vi "sweep_finished.vi"(8 "error in (no error)":errorcluster, 11 "DataCollectionMG091001IntrinsicImaging in":refnum<class "DataCollectionMG091001IntrinsicImaging.lvclass">) -> (0 "error out":errorcluster, 3 "DataCollectionMG091001IntrinsicImaging out":refnum<class "DataCollectionMG091001IntrinsicImaging.lvclass">)   [LabVIEW 2010, in "DataCollectionMG091001IntrinsicImaging.lvclass"]
uses:
  DataCollectionMG091001IntrinsicImaging.lvclass
  DataCollectionMG091001IntrinsicImaging.lvclass/DataCollectionMG091001IntrinsicImaging.ctl
  ExperimentController/GenericExperimentController/GenericExperimentController/trigger_enum.ctl
  ExperimentController/GenericExperimentController/GenericExperimentController/GenericExperimentController.lvclass
  common/classes/GenericComponent/GenericComponent/class_data.vi
  common/classes/GenericComponent/GenericComponent/GenericComponent.lvclass
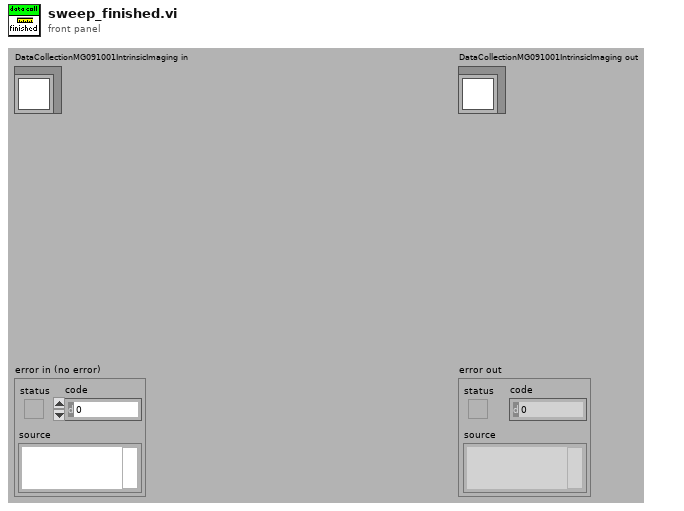
[diagram p1: front panel]
types:
  T1 = typedef "GenericExperimentController.lvclass/trigger_enum.ctl" = enum16{"NULL", "proceed", "prepare"}
  T2 = typedef "DataCollectionMG091001IntrinsicImaging.lvclass/individual_sweeps_saving_enum.ctl" = enum32{"autosave sweeps on the fly", "save individual sweeps", "don't save individual sweeps"}
  T3 = typedef "run_mode_enum.ctl" = enum16{"focus mode", "single sweep mode", "experiment mode"}
  T4 = typedef "main_trigger_enum.ctl" = enum16{"NULL", "initialise", "terminate", "start", "stop", "change objective", "change experimentController", "change imagingMode", "save notebook", "started saving", "finished saving", "expCtr ready", "expCtr missing", "imgMd ready", "imgMd missing", "scanHd ready", "scanHd missing", "DAQ ready", "DAQ missing", "imgAsm ready", "imgAsm missing", "dataColl ready", "dataColl missing", "display ready", "display missing", "analysr ready", "analysr missing", "instrmnt ready", "instrmnt missing", "stimltr ready", "stimltr missing", "stage ready", "stage missing"}
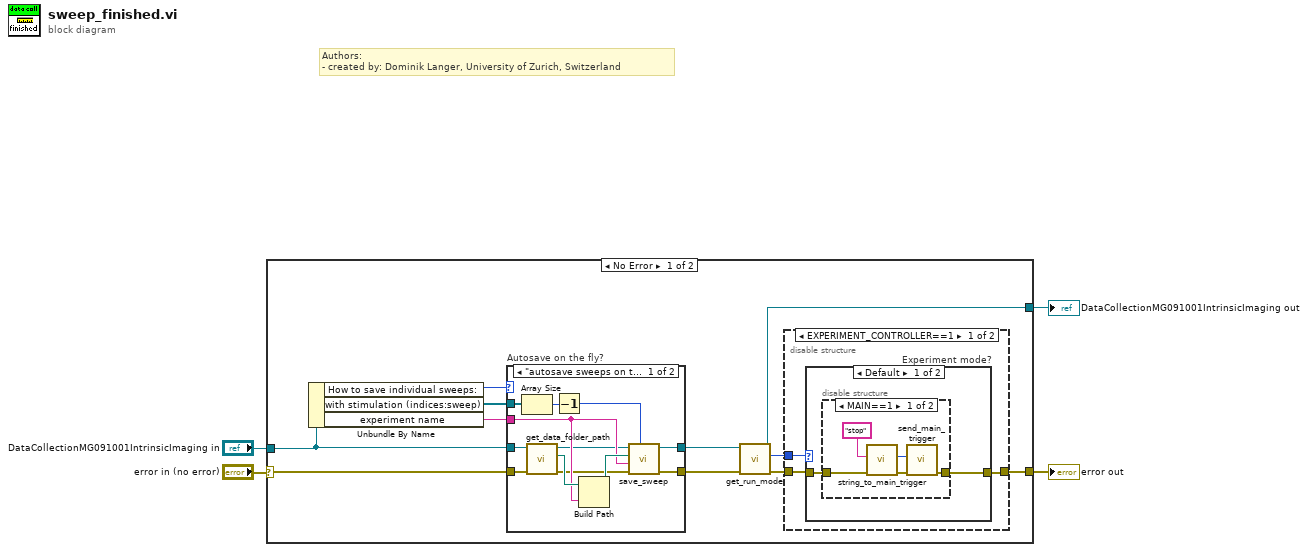
[diagram p0: block diagram]
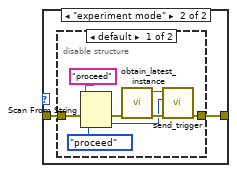
[diagram p3: hidden frame]
diagram:
  # "Authors: \n- created by: Dominik Langer, University of Zurich, Switzerland"
  n1 = case shown="No Error" "error in (no error)" {
    selector: "error in (no error)" -> [w11 w53]
    tunnel: "DataCollectionMG091001IntrinsicImaging in" -> [w12 w54]
    tunnel: [w8 w53] -> w2
    tunnel: [w5 w54] -> w1
    frame No Error {
      n2 = Unbundle By Name(w12) -> ("How to save individual sweeps:"=w13:T2, "with stimulation (indices:sweep)"=w14:refnum<class "ImageCollection.lvclass">[], "experiment name"=w15:string)
      n3 = case "Autosave on the fly?" shown="\"autosave sweeps on the fly\"" w13 {
        tunnel: [w50 w52] -> w6
        tunnel: [w49 w51] -> w7
        tunnel: w12 -> [w48 w52]
        tunnel: w11 -> [w47 w51]
        tunnel: w15 -> [w44 _]
        tunnel: w14 -> [w41 _]
        frame "autosave sweeps on the fly" {
          n4 = Array Size(array=w41) -> (size(s)=w40:i32)
          n5 = call-dynamic "get_data_folder_path.vi"("error in (no error)"=w47, "GenericComponent in"=w48) -> ("error out"=w43:errorcluster, "data folder path"=w46:path, "GenericComponent out"=w42:refnum<class "DataCollectionMG091001IntrinsicImaging.lvclass">)  [unwired: 7 in]
          n6 = Decrement(x=w40) -> (x-1=w39:i32)
          n7 = Build Path(base path=w46, name or relative path=w44) -> (appended path=w45:path)
          n8 = call-dynamic "save_sweep.vi"("sweep index"=w39, "error in (no error)"=w43, "base name"=w44, "folder path"=w45, "DataCollectionMG091001IntrinsicImaging in"=w42) -> ("error out"=w49:errorcluster, "DataCollectionMG091001IntrinsicImaging out"=w50:refnum<class "DataCollectionMG091001IntrinsicImaging.lvclass">)  [unwired: 5 in]
        }
        frame Default {
        }
      }
      n9 = call "get_run_mode.vi"("error in (no error)"=w7, "GenericPlugin in"=w6) -> ("error out"=w9:errorcluster, "run mode"=w10:T3, "GenericPlugin out"=w5:refnum<class "DataCollectionMG091001IntrinsicImaging.lvclass">)  [unwired: 5 in, 2 out]
      n10 = disable-structure shown="EXPERIMENT_CONTROLLER==1" {
        disable-tunnel: w9 -> [w16 w38]
        disable-tunnel: [w18 w38] -> w8
        disable-tunnel: w10 -> [w17 _]
        frame condition #0 (active) {
          n11 = case "Experiment mode?" shown="Default" w17 {
            tunnel: [w20 w27] -> w18
            tunnel: w16 -> [w19 w28]
            frame Default {
              n12 = disable-structure shown="MAIN==1" {
                disable-tunnel: [w25 w26] -> w20
                disable-tunnel: w19 -> [w24 w26]
                frame condition #0 (active) {
                  n13 = call "string_to_main_trigger.vi"("error in (no error)"=w24, "trigger string"="stop") -> ("error out"=w22:errorcluster, "main trigger"=w23:T4)  [unwired: 8 in]
                  n14 = call "send_main_trigger.vi"("error in (no error)"=w22, "trigger"=w23) -> ("error out"=w25:errorcluster)  [unwired: 9 in]
                }
                frame condition #1 {
                }
              }
            }
            frame "experiment mode" {
              n15 = disable-structure shown="default" {
                disable-tunnel: w28 -> [w32 w37]
                disable-tunnel: [w36 w37] -> w27
                frame condition #0 (active) {
                  n16 = Scan From String(input string="proceed", error in=w32, default 1=trigger_enum."proceed" ("trigger")) -> (error out=w31:errorcluster, output 1=w30:T1)  [unwired: 2 in, 2 out]
                  n17 = call "obtain_latest_instance.vi"("error in (no error)"=w31) -> ("error out"=w35:errorcluster, "GenericExperimentController out"=w34:refnum<class "GenericExperimentController.lvclass">)  [unwired: 1 in, 8 out]
                  n18 = call-dynamic "send_trigger.vi"("error in (no error)"=w35, "trigger"=w30, "GenericExperiment in"=w34) -> ("error out"=w36:errorcluster)  [unwired: 8 out]
                }
                frame condition #1 {
                }
              }
            }
          }
        }
        frame condition #1 {
        }
      }
    }
    frame Error {
    }
  }
  "error out" <- w2
  "DataCollectionMG091001IntrinsicImaging out" <- w1
